vi "FileIO_Parse_ERD_JSON.vi"(0 "ERD JSON File":path, 11 "Error In":errorcluster) -> (4 "ERD Names":string[](array[string]), 6 "ERD Numbers":u16[](array[numeric]) format="%.0x", 8 "#ERDs Found":i32, 15 "Error Out":errorcluster)   [LabVIEW 2019]
panel:
  out "Array":string[](array[string])
  out "ERD Name":string
  in  "ERD Number":u16 format="%x"
  out "ERDLisrAll":T1(array[cluster]) {"ERD Number" format="%x"}
  in  "Cluster 2":T2
  out "JSON Data":T3
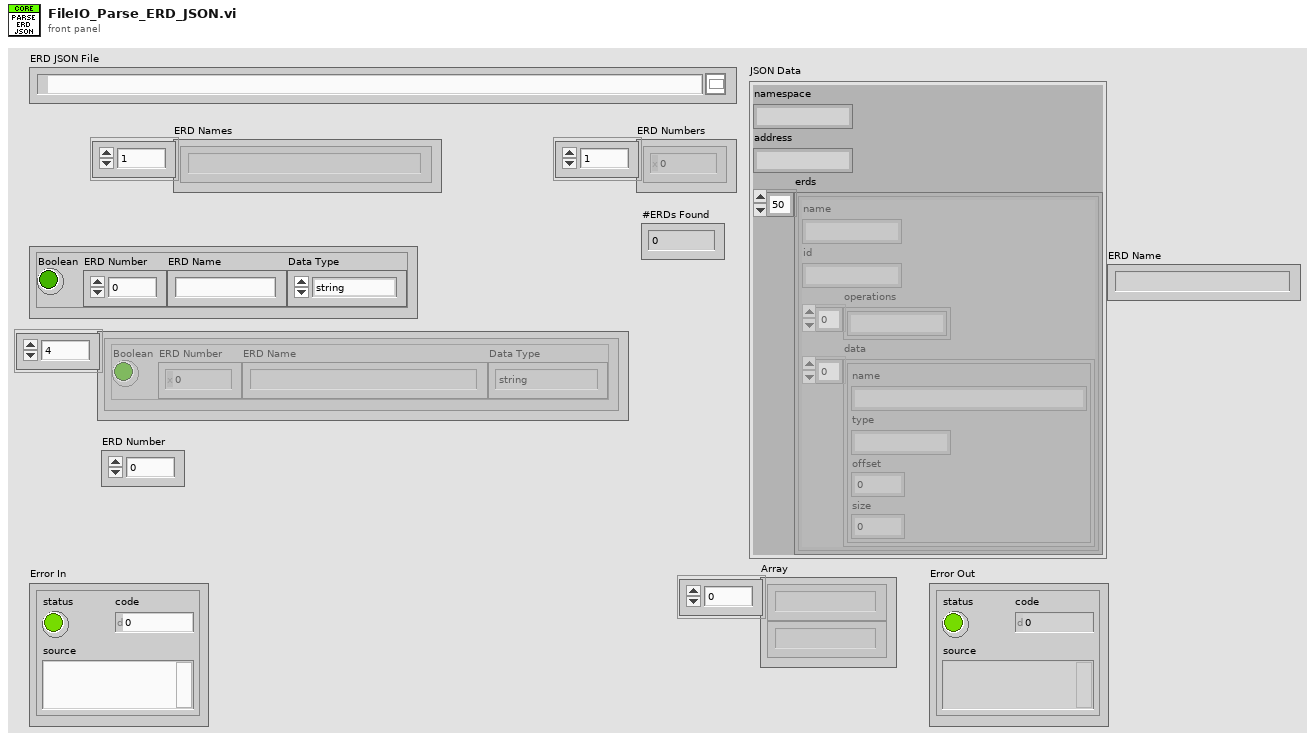
[diagram p1: front panel]
types:
  T1 = cluster{"Boolean":bool, "ERD Number":u16, "ERD Name":string, "Data Type":enum16{"string", "boolean", "uint8_t", "uint16_t", "uint32_t", "uint64_t"}}[]
  T2 = cluster{"Boolean":bool, "ERD Number":u16, "ERD Name":string, "Data Type":enum16{"string", "boolean", "uint8_t", "uint16_t", "uint32_t", "uint64_t"}}
  T3 = cluster{"namespace":string, "address":string, "erds":cluster{"name":string, "id":string, "operations":string[], "data":cluster{"name":string, "type":string, "offset":i32, "size":i32}[]}[]}
  T4 = enum16{"string", "boolean", "uint8_t", "uint16_t", "uint32_t", "uint64_t"}
  T5 = cluster{"name":string, "id":string, "operations":string[], "data":cluster{"name":string, "type":string, "offset":i32, "size":i32}[]}[]
  T6 = cluster{"name":string, "type":string, "offset":i32, "size":i32}[]
  T7 = cluster{"name":string, "type":string, "offset":i32, "size":i32}
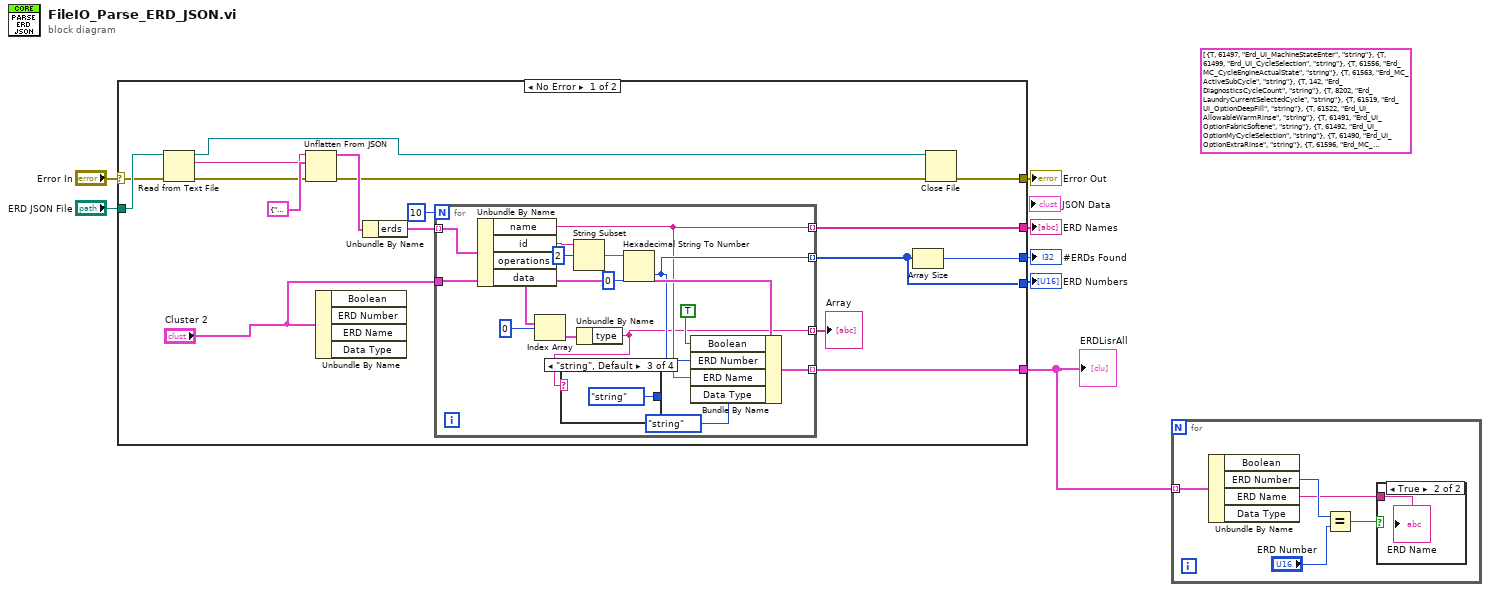
[diagram p0: block diagram]
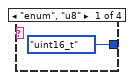
[diagram p3: hidden frame]
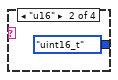
[diagram p4: hidden frame]
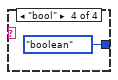
[diagram p5: hidden frame]
diagram:
  (unwired) T1 [{"Boolean"=TRUE, "ERD Number"=61497, "ERD Name"="Erd_UI_MachineStateEnter", "Data Type"=enum."string"}, {"Boolean"=TRUE, "ERD Number"=61499, "ERD Name"="Erd_UI_CycleSelection", "Data Type"=enum."string"}, {"Boolean"=TRUE, "ERD Number"=61556, "ERD Name"="Erd_MC_CycleEngineActualState", "Data Type"=enum."string"}, {"Boolean"=TRUE, "ERD Number"=61563, "ERD Name"="Erd_MC_ActiveSubCycle", "Data Type"=enum."string"}, {"Boolean"=TRUE, "ERD Number"=142, "ERD Name"="Erd_DiagnosticsCycleCount", "Data Type"=enum."string"}, {"Boolean"=TRUE, "ERD Number"=8202, "ERD Name"="Erd_LaundryCurrentSelectedCycle", "Data Type"=enum."string"}, {"Boolean"=TRUE, "ERD Number"=61519, "ERD Name"="Erd_UI_OptionDeepFill", "Data Type"=enum."string"}, {"Boolean"=TRUE, "ERD Number"=61522, "ERD Name"="Erd_UI_AllowableWarmRinse", "Data Type"=enum."string"}, {"Boolean"=TRUE, "ERD Number"=61491, "ERD Name"="Erd_UI_OptionFabricSoftene", "Data Type"=enum."string"}, {"Boolean"=TRUE, "ERD Number"=61492, "ERD Name"="Erd_UI_OptionMyCycleSelection", "Data Type"=enum."string"}, {"Boolean"=TRUE, "ERD Number"=61490, "ERD Name"="Erd_UI_OptionExtraRinse", "Data Type"=enum."string"}, {"Boolean"=TRUE, "ERD Number"=61596, "ERD Name"="Erd_MC_WaterValvesActualState", "Data Type"=enum."string"}, {"Boolean"=TRUE, "ERD Number"=61594, "ERD Name"="Erd_MC_DrainPumpActualState", "Data Type"=enum."string"}, {"Boolean"=TRUE, "ERD Number"=61561, "ERD Name"="Erd_MC_RecirculationPumpState.testModeEnabled", "Data Type"=enum."string"}, {"Boolean"=TRUE, "ERD Number"=61551, "ERD Name"="Erd_MC_LidSwitchState", "Data Type"=enum."string"}, {"Boolean"=TRUE, "ERD Number"=61630, "ERD Name"="Erd_Drive_MotorEnableActualState", "Data Type"=enum."string"}, {"Boolean"=TRUE, "ERD Number"=61595, "ERD Name"="Erd_MC_WaterValveEnableActualStat", "Data Type"=enum."string"}, {"Boolean"=TRUE, "ERD Number"=61632, "ERD Name"="Erd_Drive_ModeShiftMotorState", "Data Type"=enum."string"}, {"Boolean"=TRUE, "ERD Number"=61631, "ERD Name"="Erd_Drive_ModeShiftFeedbackStat", "Data Type"=enum."string"}, {"Boolean"=TRUE, "ERD Number"=61577, "ERD Name"="Erd_MC_ChildSafetyStatus", "Data Type"=enum."string"}, {"Boolean"=TRUE, "ERD Number"=61495, "ERD Name"="Erd_UI_OptionWaterTemperature", "Data Type"=enum."string"}, {"Boolean"=TRUE, "ERD Number"=8213, "ERD Name"="Erd_UI_OptionSoilLevel", "Data Type"=enum."string"}, {"Boolean"=TRUE, "ERD Number"=61493, "ERD Name"="Erd_UI_OptionSpinLevel", "Data Type"=enum."string"}, {"Boolean"=TRUE, "ERD Number"=61496, "ERD Name"="Erd_UI_OptionLoadSize", "Data Type"=enum."string"}, {"Boolean"=TRUE, "ERD Number"=8208, "ERD Name"="Erd_DelayStartTimeInMinutesPublic", "Data Type"=enum."string"}, {"Boolean"=TRUE, "ERD Number"=61554, "ERD Name"="Erd_MC_LidLockRequestState", "Data Type"=enum."string"}, {"Boolean"=TRUE, "ERD Number"=61515, "ERD Name"="Erd_UI_OptionAutoSoakLevel", "Data Type"=enum."string"}, {"Boolean"=TRUE, "ERD Number"=61603, "ERD Name"="Erd_Drive_DryLoadSizeInLbsQ5", "Data Type"=enum."string"}, {"Boolean"=TRUE, "ERD Number"=61544, "ERD Name"="Erd_MC_WetLoadGallons", "Data Type"=enum."string"}, {"Boolean"=TRUE, "ERD Number"=61549, "ERD Name"="Erd_MC_WetLoadGallons", "Data Type"=enum."string"}, {"Boolean"=TRUE, "ERD Number"=61550, "ERD Name"="Erd_MC_LoadType", "Data Type"=enum."string"}, {"Boolean"=TRUE, "ERD Number"=61565, "ERD Name"="Erd_MC_TargetLevelInInchesOfWaterx100Erd_MC_TargetLevelInInchesOfWaterx1000", "Data Type"=enum."string"}, {"Boolean"=TRUE, "ERD Number"=61537, "ERD Name"="Erd_RemainingCycleTimeInSeconds", "Data Type"=enum."string"}, {"Boolean"=TRUE, "ERD Number"=1, "ERD Name"="Erd_UnitSkuNumber", "Data Type"=enum."string"}, {"Boolean"=TRUE, "ERD Number"=61608, "ERD Name"="Erd_Drive_SpeedSensorShaft", "Data Type"=enum."string"}, {"Boolean"=TRUE, "ERD Number"=61609, "ERD Name"="Erd_SpeedSensorReadingForTestLoop", "Data Type"=enum."string"}, {"Boolean"=TRUE, "ERD Number"=61611, "ERD Name"="Erd_Drive_LoadCurrentRms", "Data Type"=enum."string"}, {"Boolean"=TRUE, "ERD Number"=61545, "ERD Name"="Erd_MC_CurrentTubInGallonsx100", "Data Type"=enum."string"}, {"Boolean"=TRUE, "ERD Number"=65314, "ERD Name"="Erd_Drive_ModeShiftActualState", "Data Type"=enum."string"}, {"Boolean"=TRUE, "ERD Number"=61555, "ERD Name"="Erd_MC_LidLockActualState", "Data Type"=enum."string"}, {"Boolean"=TRUE, "ERD Number"=61568, "ERD Name"="Erd_MC_LidLockFeedbackState", "Data Type"=enum."string"}, {"Boolean"=TRUE, "ERD Number"=61623, "ERD Name"="Erd_Drive_CycleEngineActualState", "Data Type"=enum."string"}, {"Boolean"=TRUE, "ERD Number"=61617, "ERD Name"="Erd_Drive_MotorMode", "Data Type"=enum."string"}, {"Boolean"=TRUE, "ERD Number"=61559, "ERD Name"="Erd_MC_WaterTemperature", "Data Type"=enum."string"}, {"Boolean"=FALSE, "ERD Number"=0, "ERD Name"="", "Data Type"=enum."string"}, {"Boolean"=TRUE, "ERD Number"=2, "ERD Name"="Erd_UnitSerialNumber", "Data Type"=enum."string"}] ("ERDListAll")
  n1 = case shown="No Error" "Error In" {
    selector: "Error In" -> [w22 w44]
    tunnel: "ERD JSON File" -> [w23 _]
    tunnel: [w24 _] -> w6
    tunnel: [w13 _] -> w5
    tunnel: [w12 _] -> w4
    tunnel: [w21 w44] -> w3
    tunnel: [w10 _] -> w1
    frame No Error {
      n2 = Read from Text File(file (use dialog)=w23, error in=w22) -> (refnum out=w14:refnum<file>, text=w17:string, error out=w16:errorcluster)  [unwired: 2 in, 1 out]
      n3 = Unflatten From JSON(JSON string=w17, type and defaults=T3 {"namespace"="", "address"="", "erds"=[]}, error in (no error)=w16) -> (value=w19:T3, error out=w15:errorcluster)  [unwired: 4 in]
      n4 = Unbundle By Name("Cluster 2") -> ()  [unwired: 4 out]
      n5 = Unbundle By Name(w19) -> ("erds"=w18:T5)
      n6 = for {
        N: 10 -> [_]
        tunnel: w18 -> [w39] mode=indexing
        tunnel: [w31] -> w13 mode=indexing
        tunnel: [w32] -> w12 mode=indexing
        tunnel: "Cluster 2" -> [w34]
        tunnel: [w27] -> w10 mode=indexing
        tunnel: [w26] -> w8 mode=indexing
        n7 = Unbundle By Name(w39) -> ("name"=w31:string, "id"=w38:string, "data"=w30:T6)  [unwired: 1 out]
        n8 = Index Array(array=w30, index=0) -> (element=w28:T7)
        n9 = String Subset(string=w38, offset (0)=2) -> (substring=w36:string)  [unwired: 1 in]
        n10 = Unbundle By Name(w28) -> ("type"=w26:string)
        n11 = case shown="\"string\", Default" w26 {
          tunnel: [T4."uint16_t" ("Data Type") T4."uint16_t" ("Data Type") T4."string" ("Data Type") T4."boolean" ("Data Type")] -> _
          frame "enum", "u8" {
          }
          frame "u16" {
          }
          frame "string", Default {
          }
          frame "bool" {
          }
        }
        n12 = Hexadecimal String To Number(string=w36, default (0uL)=u16 0 ("default (0 U32)")) -> (number=w32:u16)  [unwired: 1 in, 1 out]
        n13 = Bundle By Name(cluster=w34, "Boolean"=TRUE, "ERD Number"=w32, "ERD Name"=w31, "Data Type"=T4."string") -> (w27:T2)
      }
      "Array" <- w8
      n14 = Array Size(array=w12) -> (size(s)=w24:i32)
      n15 = Close File(refnum=w14, error in=w15) -> (error out=w21:errorcluster)  [unwired: 1 out]
    }
    frame Error {
    }
  }
  "#ERDs Found" <- w6
  "ERD Names" <- w5
  "ERD Numbers" <- w4
  "Error Out" <- w3
  "ERDLisrAll" <- w1
  n16 = for {
    tunnel: w1 -> [w49] mode=indexing
    n17 = Unbundle By Name(w49) -> ("ERD Number"=w48:u16, "ERD Name"=w45:string)  [unwired: 2 out]
    n18 = Equal?(x=w48, y="ERD Number") -> (x = y?=w46:bool)
    n19 = case shown="True" w46 {
      tunnel: w45 -> [_ w50]
      frame False {
      }
      frame True {
        "ERD Name" <- w50
      }
    }
  }
